vi "Analog Input.vi"(6 "clai. Parmeter":T1, 8 "error in":errorcluster, 9 "Min Value":string[](array[string]), 10 "Max Value":string[](array[string]), 11 "DAQmx Analog Input Setting":T2={"DAQmx Analog Input_00"="Dev1/ai0", "DAQmx Analog Input_01"="Dev1/ai1", "DAQmx Analog Input_02"="Dev1/ai2", "DAQmx Analog Input_03"="Dev1/ai3", "DAQmx Analog Input_04"="Dev1/ai4", "DAQmx Analog Input_05"="Dev1/ai5", "DAQmx Analog Input_06"="Dev1/ai6", "DAQmx Analog Input_07"="Dev1/ai7", "DAQmx Analog Input_00 2"="Dev1/ai8", "DAQmx Analog Input_01 2"="Dev1/ai9", "DAQmx Analog Input_02 2"="Dev1/ai10", "DAQmx Analog Input_03 2"="Dev1/ai11", "DAQmx Analog Input_04 2"="Dev1/ai12", "DAQmx Analog Input_05 2"="Dev1/ai13", "DAQmx Analog Input_06 2"="Dev1/ai14", "DAQmx Analog Input_07 2"="Dev1/ai15", "DAQmx Analog Input_00 3"="Dev1/ai16", "DAQmx Analog Input_01 3"="Dev1/ai17", "DAQmx Analog Input_02 3"="Dev1/ai18", "DAQmx Analog Input_03 3"="Dev1/ai19", "DAQmx Analog Input_04 3"="Dev1/ai20", "DAQmx Analog Input_05 3"="Dev1/ai21", "DAQmx Analog Input_06 3"="Dev1/ai22", "DAQmx Analog Input_07 3"="Dev1/ai23", "DAQmx Analog Input_00 4"="Dev1/ai24", "DAQmx Analog Input_01 4"="Dev1/ai25", "DAQmx Analog Input_02 4"="Dev1/ai26", "DAQmx Analog Input_03 4"="Dev1/ai27", "DAQmx Analog Input_04 4"="Dev1/ai28", "DAQmx Analog Input_05 4"="Dev1/ai29", "DAQmx Analog Input_06 4"="Dev1/ai30", "DAQmx Analog Input_07 4"="Dev1/ai31"}) -> (0 "error out":errorcluster, 1 "Exit":bool)   [LabVIEW 2015]
uses:
  <vilib>/DAQmx/read.llb/DAQmx Read (Analog 2D DBL NChan NSamp).vi
  <vilib>/DAQmx/create/channels.llb/DAQmx Create Channel (AI-Voltage-Basic).vi
  <vilib>/DAQmx/configure/timing.llb/DAQmx Timing (Sample Clock).vi
  Galobal variable_TI.vi
  <vilib>/DAQmx/miscellaneous.llb/DAQmx Fill In Error Info.vi
panel:
  out "x-y":u32
  out "error out 2":errorcluster
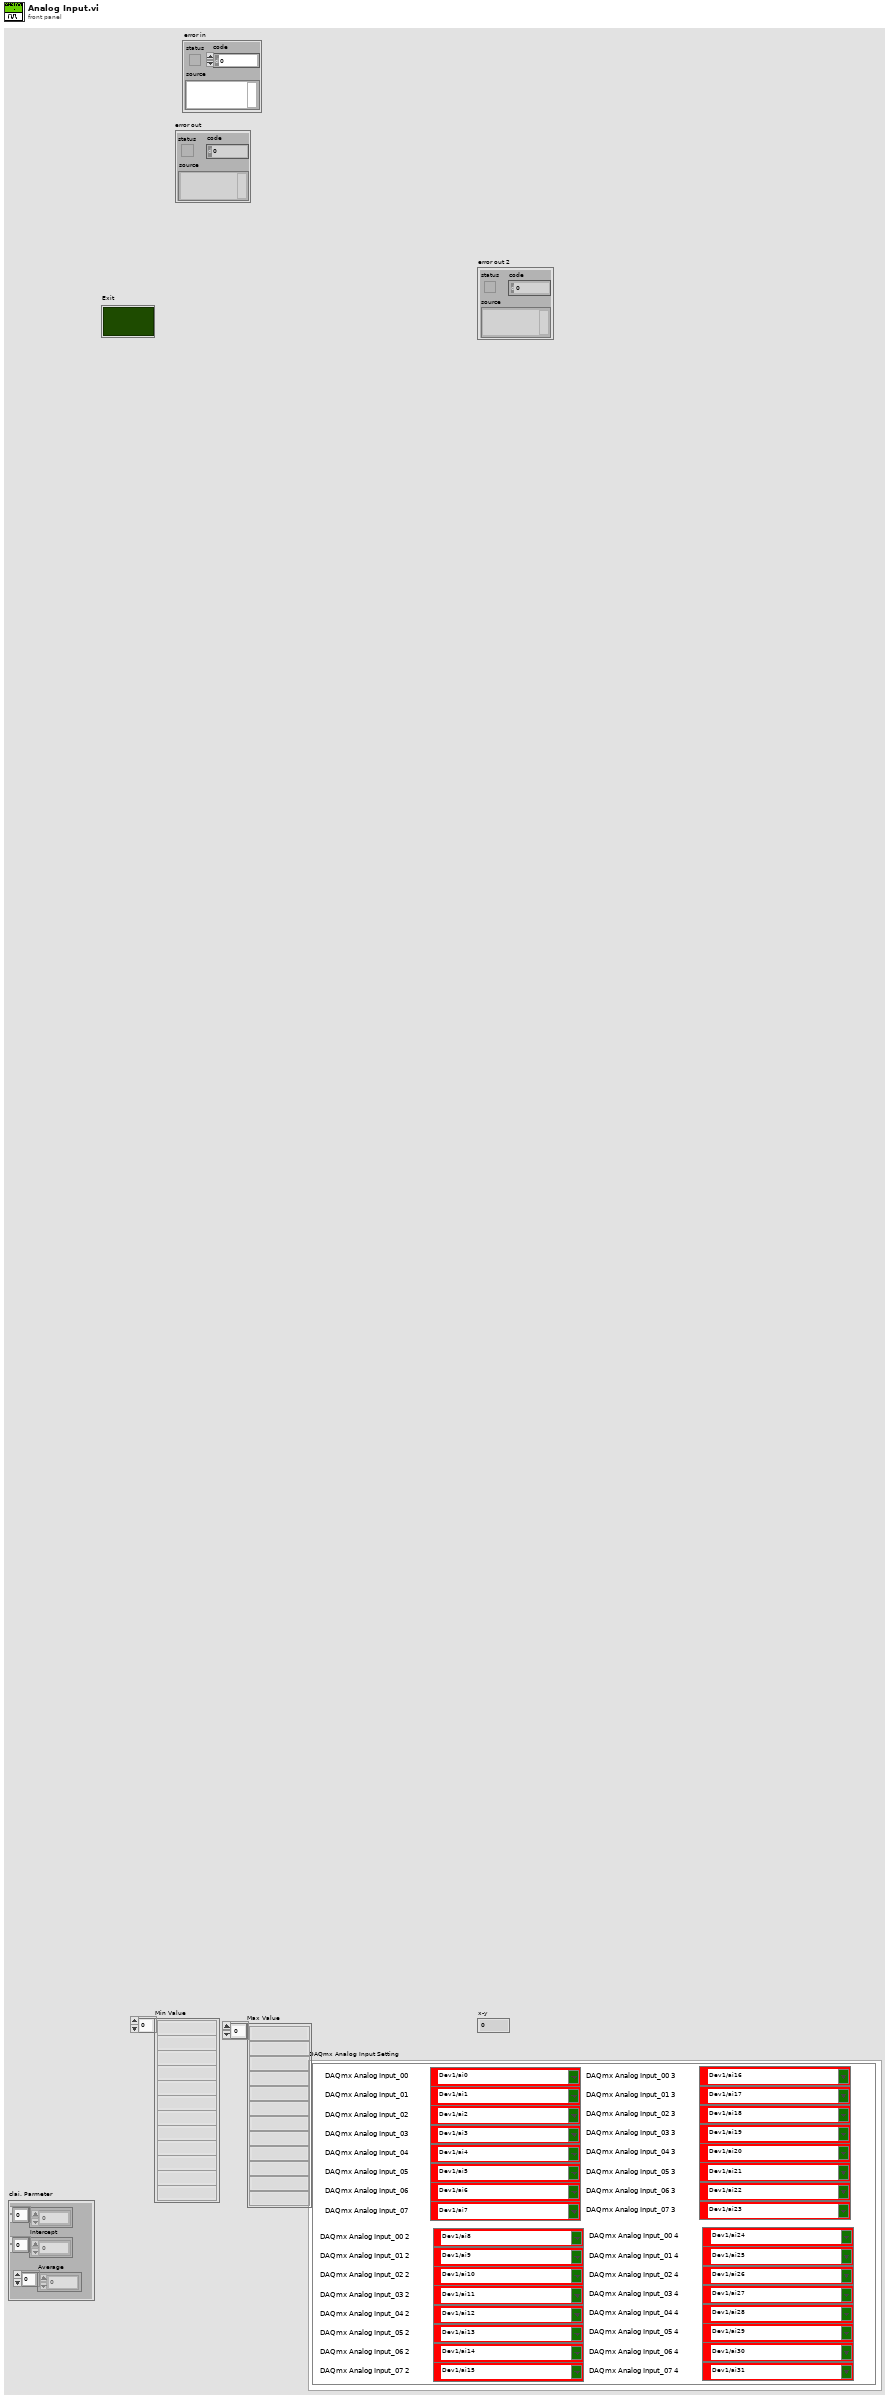
[diagram p1: front panel]
types:
  T1 = cluster{"Slop":dbl[], "Intercept":dbl[], "Average ":i16[]}
  T2 = cluster{"DAQmx Analog Input_00":tag, "DAQmx Analog Input_01":tag, "DAQmx Analog Input_02":tag, "DAQmx Analog Input_03":tag, "DAQmx Analog Input_04":tag, "DAQmx Analog Input_05":tag, "DAQmx Analog Input_06":tag, "DAQmx Analog Input_07":tag, "DAQmx Analog Input_00 2":tag, "DAQmx Analog Input_01 2":tag, "DAQmx Analog Input_02 2":tag, "DAQmx Analog Input_03 2":tag, "DAQmx Analog Input_04 2":tag, "DAQmx Analog Input_05 2":tag, "DAQmx Analog Input_06 2":tag, "DAQmx Analog Input_07 2":tag, "DAQmx Analog Input_00 3":tag, "DAQmx Analog Input_01 3":tag, "DAQmx Analog Input_02 3":tag, "DAQmx Analog Input_03 3":tag, "DAQmx Analog Input_04 3":tag, "DAQmx Analog Input_05 3":tag, "DAQmx Analog Input_06 3":tag, "DAQmx Analog Input_07 3":tag, "DAQmx Analog Input_00 4":tag, "DAQmx Analog Input_01 4":tag, "DAQmx Analog Input_02 4":tag, "DAQmx Analog Input_03 4":tag, "DAQmx Analog Input_04 4":tag, "DAQmx Analog Input_05 4":tag, "DAQmx Analog Input_06 4":tag, "DAQmx Analog Input_07 4":tag}
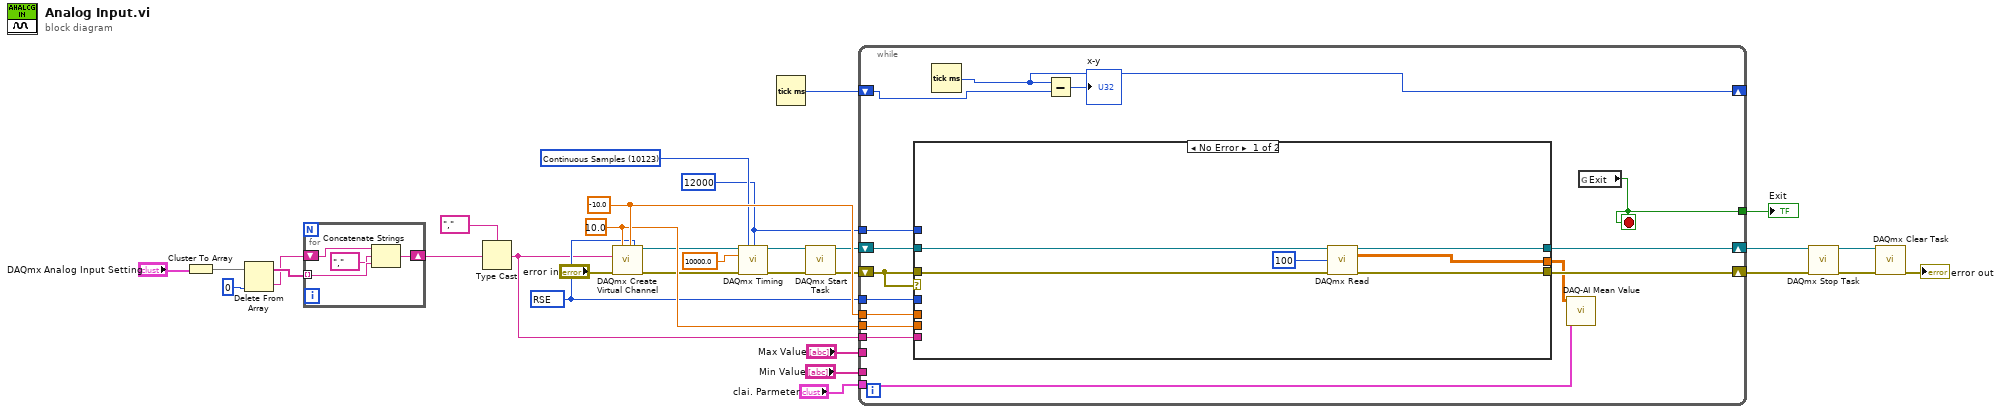
[diagram p0: block diagram]
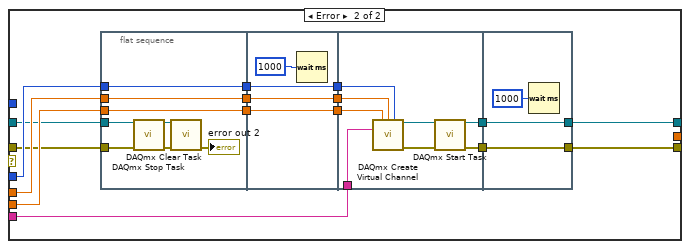
[diagram p2: hidden frame]
diagram:
  w8 = 12000 ("samples per channel")
  w23 = 10123 items=["Finite Samples"=10178, "Continuous Samples"=10123, "Hardware Timed Single Point"=12522] ("sample mode")
  w29 = 10083 items=["default"=-1, "RSE"=10083, "NRSE"=10078, "Differential"=10106, "Pseudodifferential"=12529] ("input terminal configuration")
  w31 = -10.0 ("minimum value")
  w30 = 10.0 ("maximum value")
  n1 = Cluster To Array(cluster="DAQmx Analog Input Setting") -> (array=w20:tag[])
  n2 = Delete From Array(array=w20, index=0) -> (deleted portion=w17:tag, array with subset deleted=w19:tag[])  [unwired: 1 in]
  n3 = for {
    tunnel: w19 -> [w35] mode=indexing
    shift-right: [w33] -> w15
    shift-left: w17 -> [w32]
    n4 = Concatenate Strings(w32, tag "," ("1."), w35) -> (w33:string)
  }
  n5 = Type Cast(type=tag "," ("1."), x=w15) -> (*(type *) &x=w21:tag)
  n6 = call-poly <vilib>:"DAQmx Create Virtual Channel.vi"("maximum value"=w30, "minimum value"=w31, "input terminal configuration"=w29, "physical channels"=w21, "error in"="error in") -> ("task out"=w27:refnum<k21>, "error out"=w26:errorcluster)  [unwired: 4 in, 5 out]
  n7 = call-poly <vilib>:"DAQmx Timing.vi"("task/channels in"=w27, "sample mode"=w23, "samples per channel"=w8, "rate"=10000.0, "error in"=w26) -> ("task out"=w25:refnum<k21>, "error out"=w24:errorcluster)  [unwired: 9 in]
  n8 = Tick Count (ms)() -> (millisecond timer value=w7:u32)
  n9 = call <vilib>:"DAQmx Start Task.vi"("task/channels in"=w25, "error in"=w24) -> ("task out"=w13:refnum<k21>, "error out"=w12:errorcluster)  [unwired: 12 out]
  n10 = while {
    shift-right: [w47] -> w11
    shift-left: w12 -> [w50]
    shift-right: [w48] -> w10
    shift-left: w13 -> [w49]
    tunnel: w21 -> [w46]
    tunnel: w31 -> [w45]
    tunnel: w30 -> [w44]
    tunnel: w29 -> [w43]
    tunnel: [w41] -> w9
    tunnel: w8 -> [w40]
    shift-right: [w38] -> _
    shift-left: w7 -> [w39]
    tunnel: "Max Value" -> [_]
    tunnel: "Min Value" -> [_]
    tunnel: "clai. Parmeter" -> [w36]
    stop <- w41 stop-if-true
    n11 = case shown="No Error" w50 {
      tunnel: w50 -> [w55 w59]
      tunnel: w49 -> [w56 w60]
      tunnel: [w54 w58] -> w48
      tunnel: [w53 w57] -> w47
      tunnel: w46 -> [_ w72]
      tunnel: w45 -> [_ w71]
      tunnel: w44 -> [_ w70]
      tunnel: w43 -> [_ w69]
      tunnel: [w52 _] -> w42
      tunnel: w40 -> [_ _]
      frame No Error {
        n12 = call-poly <vilib>:"DAQmx Read.vi"("task/channels in"=w56, "number of samples per channel"=100, "error in"=w55) -> ("task out"=w54:refnum<k21>, "data"=w52:dbl[][], "error out"=w53:errorcluster)  [unwired: 10 out]
      }
      frame Error {
        n13 = flat-sequence {
          tunnel: w69 -> [w78]
          tunnel: w70 -> [w79]
          tunnel: w71 -> [w80]
          tunnel: [w80] -> w63
          tunnel: [w79] -> w62
          tunnel: [w78] -> w61
          tunnel: w60 -> [w76]
          tunnel: w59 -> [w75]
          tunnel: [w84] -> w66
          tunnel: [w83] -> w65
          tunnel: [w82] -> w64
          tunnel: w63 -> [w84]
          tunnel: w62 -> [w83]
          tunnel: w61 -> [w82]
          tunnel: w72 -> [w90]
          tunnel: [w86] -> w68
          tunnel: [w85] -> w67
          tunnel: w66 -> [w89]
          tunnel: w65 -> [w88]
          tunnel: w64 -> [w87]
          tunnel: [w94] -> w57
          tunnel: [w95] -> w58
          tunnel: w68 -> [w95]
          tunnel: w67 -> [w94]
          frame #0 {
            n14 = call <vilib>:"DAQmx Stop Task.vi"("task/channels in"=w76, "error in"=w75) -> ("task out"=w73:refnum<k21>, "error out"=w77:errorcluster)  [unwired: 12 in]
            n15 = call <vilib>:"DAQmx Clear Task.vi"("task in"=w73, "error in"=w77) -> ("error out"=→"error out 2":errorcluster)  [unwired: 13 in]
          }
          frame #1 {
            n16 = Wait (ms)(milliseconds to wait=u32 1000) -> ()  [unwired: 1 out]
          }
          frame #2 {
            n17 = call-poly <vilib>:"DAQmx Create Virtual Channel.vi"("maximum value"=w88, "minimum value"=w89, "input terminal configuration"=w87, "physical channels"=w90) -> ("task out"=w92:refnum<k21>, "error out"=w91:errorcluster)  [unwired: 5 in, 5 out]
            n18 = call <vilib>:"DAQmx Start Task.vi"("task/channels in"=w92, "error in"=w91) -> ("task out"=w86:refnum<k21>, "error out"=w85:errorcluster)  [unwired: 12 out]
          }
          frame #3 {
            n19 = Wait (ms)(milliseconds to wait=u32 1000) -> ()  [unwired: 1 out]
          }
        }
      }
    }
    n20 = Tick Count (ms)() -> (millisecond timer value=w38:u32)
    n21 = Subtract(x=w38, y=w39) -> (x-y=→"x-y":u32)
    n22 = call "DAQ-AI Mean Value.vi"("Cluster"=w36, "data"=w42) -> ()  [unwired: 9 in, 1 out]
    n23 = global read "Galobal variable_TI.vi" "Exit"() -> (w41:bool)
  }
  "Exit" <- w9
  n24 = call <vilib>:"DAQmx Stop Task.vi"("task/channels in"=w10, "error in"=w11) -> ("task out"=w4:refnum<k21>, "error out"=w3:errorcluster)  [unwired: 12 in]
  n25 = call <vilib>:"DAQmx Clear Task.vi"("task in"=w4, "error in"=w3) -> ("error out"=→"error out":errorcluster)  [unwired: 13 in]
